vi "Pre-lim Current Detection.vi"(6 "Barcodes in":string[](array[string]), 8 "error in (no error)":errorcluster, 10 "Stop Program":bool, 11 "BoardHandle in":T1) -> (0 "error out":errorcluster, 1 "Actual Current Limit (nA) 4":dbl format="%#_13g", 2 "Actual Current Limit (nA) 3":dbl format="%#_13g", 3 "Actual Current Limit (nA) 2":dbl format="%#_13g", 4 "BoardHandle out 3":T1, 5 "Actual Current Limit (nA)":dbl format="%#_13g", 7 "Power Supply Trip":bool, 9 "Actual Voltage Level (V)":dbl format="%#_13g")   [LabVIEW 2020]
uses:
  <instrlib>/CAEN PSM/CAEN PSM.lvlib
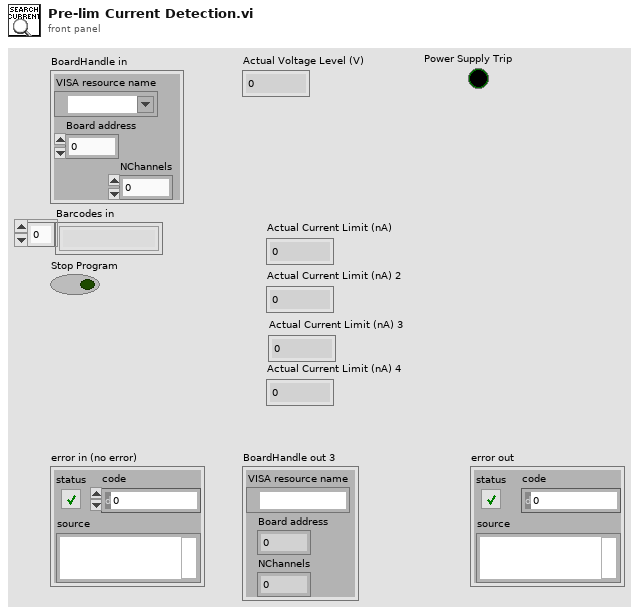
[diagram p1: front panel]
types:
  T1 = cluster{"VISA resource name":refnum<visa-resource-name>, "Board address":u8, "NChannels":u8}
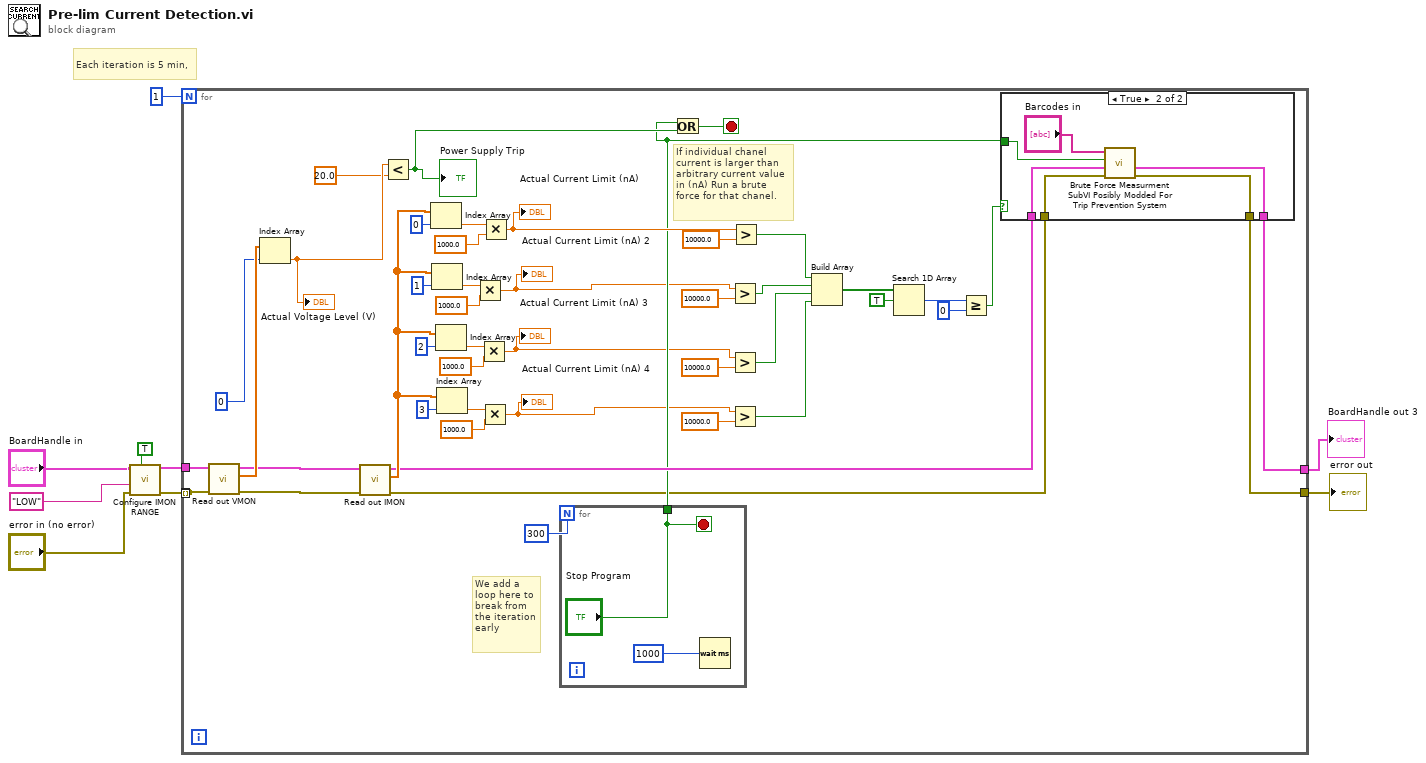
[diagram p0: block diagram]
diagram:
  # "Each iteration is 5 min,"
  n1 = call <instrlib>:"Configure IMON RANGE.vi"("All Channels (F)"=TRUE, "error in (no error)"="error in (no error)", "IMon range (LOW)"="LOW", "BoardHandle"="BoardHandle in") -> ("error out"=w6:errorcluster, "BoardHandle out"=w5:T1)  [unwired: 6 in]
  n2 = for {
    N: 1 ("N") -> [_]
    tunnel: w6 -> [w45]
    tunnel: [w26] -> w2
    tunnel: [w25] -> w1
    tunnel: w5 -> [w46]
    tunnel: [w45] -> _ mode=indexing
    stop <- w49 stop-if-true
    # "If individual chanel\ncurrent is larger than\narbitrary current value\nin (nA) Run a brute \nforce for that chanel."
    # "We add a \nloop here to\nbreak from \nthe iteration\nearly"
    n3 = call <instrlib>:"Read out VMON.vi"("error in (no error)"=w45, "BoardHandle"=w46) -> ("error out"=w53:errorcluster, "VMon values (V)"=w55:dbl[], "BoardHandle out"=w54:T1)  [unwired: 7 in]
    n4 = Index Array(array=w55, index=0) -> (element=w51:dbl)
    "Actual Voltage Level (V)" <- w51
    n5 = call <instrlib>:"Read out IMON.vi"("error in (no error)"=w53, "BoardHandle"=w54) -> ("error out"=w27:errorcluster, "IMon values (uA)"=w33:dbl[], "BoardHandle out"=w29:T1)  [unwired: 6 in, 1 out]
    n6 = Less?(x=w51, y=20.0) -> (x < y?=w48:bool)
    "Power Supply Trip" <- w48
    n7 = Index Array(array=w33, index=0) -> (element=w32:dbl)
    n8 = Index Array(array=w33, index=1) -> (element=w42:dbl)
    n9 = Index Array(array=w33, index=2) -> (element=w39:dbl)
    n10 = Index Array(array=w33, index=3) -> (element=w36:dbl)
    n11 = Multiply(x=w42, y=1000.0) -> (x*y=w21:dbl)
    "Actual Current Limit (nA) 2" <- w21
    n12 = Multiply(x=w39, y=1000.0) -> (x*y=w20:dbl)
    "Actual Current Limit (nA) 3" <- w20
    n13 = Multiply(x=w36, y=1000.0) -> (x*y=w19:dbl)
    "Actual Current Limit (nA) 4" <- w19
    n14 = Multiply(x=w32, y=1000.0) -> (x*y=w31:dbl)
    "Actual Current Limit (nA)" <- w31
    n15 = for {
      N: 300 ("dt (s) in") -> [_]
      tunnel: ["Stop Program"] -> w28
      stop <- "Stop Program" stop-if-true
      n16 = Wait (ms)(milliseconds to wait=1000) -> ()  [unwired: 1 out]
    }
    n17 = Or(x=w28, y=w48) -> (x .or. y?=w49:bool)
    n18 = Greater?(x=w21, y=10000.0) -> (0:w17:bool)
    n19 = Greater?(x=w20, y=10000.0) -> (0:w16:bool)
    n20 = Greater?(x=w19, y=10000.0) -> (0:w15:bool)
    n21 = Greater?(x=w31, y=10000.0) -> (0:w18:bool)
    n22 = Build Array(w18, w17, w16, w15) -> (w14:bool[])
    n23 = Search 1D Array(1D array=w14, element=TRUE) -> (index of element=w12:i32)  [unwired: 1 in]
    n24 = Greater Or Equal?(x=w12, y=0) -> (x >= y?=w10:bool)
    n25 = case shown="True" w10 {
      tunnel: w29 -> [w56 w62]
      tunnel: w28 -> [_ w61]
      tunnel: w27 -> [w57 w60]
      tunnel: [w56 w59] -> w26
      tunnel: [w57 w58] -> w25
      frame False {
      }
      frame True {
        n26 = call "Brute Force Measurment SubVI Posibly Modded For Trip Prevention System.vi"("error in (no error)"=w60, "BoardHandle in"=w62, "Stop Program Brute Force"=w61, "Barcodes in"="Barcodes in") -> ("error out"=w58:errorcluster, "BoardHandle out"=w59:T1)  [unwired: 5 in, 1 out]
      }
    }
  }
  "error out" <- w1
  "BoardHandle out 3" <- w2
